vi "Download Web File.vi"(6 "Show File?":bool, 8 "Error In":errorcluster, 9 "timeout (10000)":i32=10000, 10 "Dest Folder":path=path "C:/", 11 "URL":string) -> (0 "Error Out":errorcluster, 1 "body":string, 2 "headers":string, 3 "File Path":path)   [LabVIEW 2021, in "Web.lvlib"]
uses:
  Web.lvlib
  <vilib>/httpClient/LabVIEWHTTPClient.lvlib
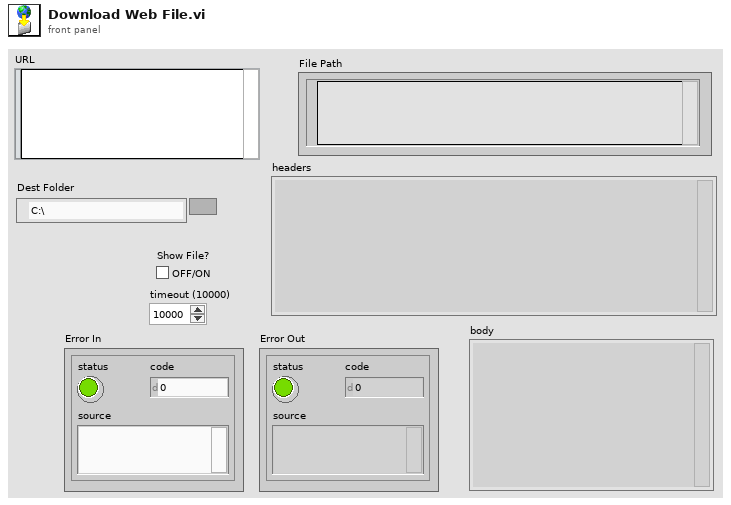
[diagram p1: front panel]
types:
  T1 = typedef "LabVIEWHTTPClient.lvlib/ClientHandle.ctl" = refnum<k1>
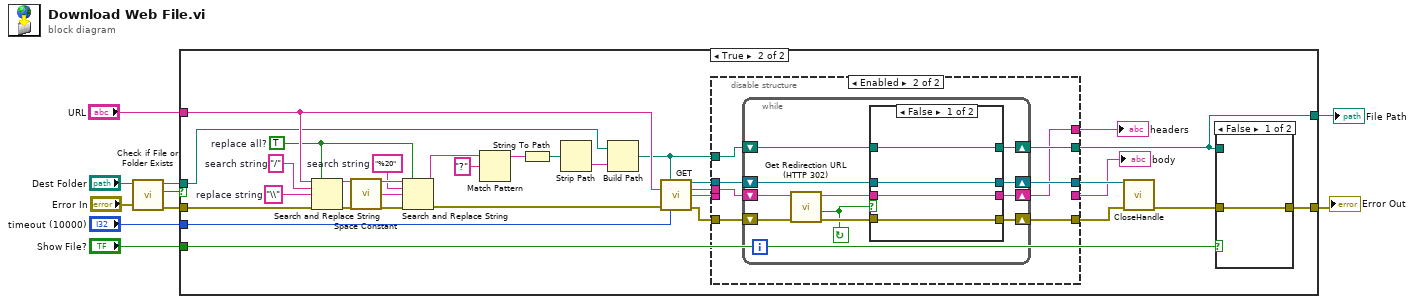
[diagram p0: block diagram]
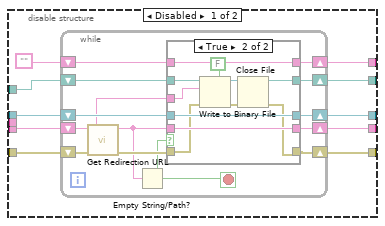
[diagram p3: hidden frame]
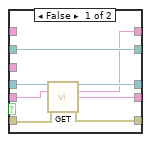
[diagram p4: hidden frame]
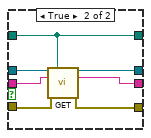
[diagram p5: hidden frame]
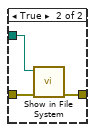
[diagram p6: hidden frame]
diagram:
  n1 = call <vilib>:"Check if File or Folder Exists.vi"("error in (no error)"="Error In", "path"="Dest Folder") -> ("error out"=w8:errorcluster, "file or folder exists?"=w5:bool, "dup path"=w7:path)  [unwired: 7 in]
  n2 = case shown="True" w5 {
    tunnel: "URL" -> [_ w41]
    tunnel: w8 -> [w11 w36]
    tunnel: w7 -> [_ w32]
    tunnel: [w11 w35] -> w2
    tunnel: "Show File?" -> [_ w34]
    tunnel: "timeout (10000)" -> [_ w33]
    tunnel: [_ w18] -> w1
    frame False {
    }
    frame True {
      w24 = "%20"  # search string
      w25 = TRUE  # replace all?
      w39 = "\\"  # replace string
      w40 = "/"  # search string
      n3 = Search and Replace String(replace all?=w25, input string=w41, search string=w40, replace string=w39, error in=w36) -> (result string=w27:string, error out=w29:errorcluster)  [unwired: 3 in, 2 out]
      n4 = call <vilib>:"Space Constant.vi"() -> ("String"=w23:string)
      n5 = Search and Replace String(replace all?=w25, input string=w27, search string=w24, replace string=w23, error in=w29) -> (result string=w26:string, error out=w28:errorcluster)  [unwired: 3 in, 2 out]
      n6 = Match Pattern(string=w26, regular expression="?") -> (before substring=w30:string)  [unwired: 1 in, 3 out]
      n7 = String To Path(string=w30) -> (path=w38:path)
      n8 = Strip Path(path=w38) -> (name=w37:string)  [unwired: 1 out]
      n9 = Build Path(base path=w32, name or relative path=w37) -> (appended path=w14:path)
      n10 = call <vilib>:"GET.vi"("output file"=w14, "url"=w41, "error in (no error)"=w28, "timeout (10000)"=w33) -> ("client handle out"=w20:T1, "headers"=w13:string, "body"=w22:string, "error out"=w21:errorcluster)  [unwired: 8 in]
      n11 = disable-structure shown="Enabled" {
        disable-tunnel: w22 -> [w51 _]
        disable-tunnel: w21 -> [w50 w91]
        disable-tunnel: w20 -> [w49 w90]
        disable-tunnel: [w48 w89] -> w19
        disable-tunnel: [w47 w88] -> w18
        disable-tunnel: [w46 w87] -> w17
        disable-tunnel: [w45 _] -> w16
        disable-tunnel: [w44 w84] -> w15
        disable-tunnel: w14 -> [w43 w86]
        disable-tunnel: w13 -> [_ w85]
        frame Disabled {
          n12 = while {
            shift-right: [w55] -> w46
            shift-left: w50 -> [w64]
            shift-right: [w58] -> w45
            shift-left: w51 -> [w57]
            shift-right: [w62] -> w48
            shift-left: w49 -> [w63]
            shift-right: [w54] -> w47
            shift-left: w43 -> [w56]
            shift-right: [w53] -> w44
            shift-left: "" -> [w52]
            stop <- w59 stop-if-true
            n13 = call "Get Redirection URL.vi"("error in (no error)"=w64, "HTTP GET Body"=w57) -> ("error out"=w61:errorcluster, "Redirection URL"=w60:string)  [unwired: 8 in]
            n14 = Empty String/Path?(string/path=w60) -> (empty?=w59:bool)
            n15 = case shown="True" w59 {
              tunnel: w63 -> [w72 w83]
              tunnel: [w71 w83] -> w62
              tunnel: w61 -> [w70 w74]
              tunnel: w60 -> [w69 w82]
              tunnel: [w68 w82] -> w58
              tunnel: w57 -> [_ w80]
              tunnel: w56 -> [w66 w81]
              tunnel: [w67 w76] -> w55
              tunnel: [w66 w75] -> w54
              tunnel: [w65 w73] -> w53
              tunnel: w52 -> [_ w73]
              frame False {
                n16 = call <vilib>:"GET.vi"("client handle"=w72, "url"=w69, "error in (no error)"=w70) -> ("client handle out"=w71:T1, "headers"=w65:string, "body"=w68:string, "error out"=w67:errorcluster)  [unwired: 9 in]
              }
              frame True {
                n17 = Write to Binary File(file (use dialog)=w81, data=w80, error in=w74, 5:FALSE ("prepend array or string size? (T)")) -> (refnum out=w78:refnum<file>, error out=w77:errorcluster)  [unwired: 2 in, 1 out]
                n18 = Close File(refnum=w78, error in=w77) -> (path=w75:path, error out=w76:errorcluster)
              }
            }
          }
        }
        frame Enabled {
          n19 = while {
            shift-right: [w94] -> w87
            shift-left: w91 -> [w102]
            shift-right: [w97] -> w84
            shift-left: w85 -> [w96]
            shift-right: [w100] -> w89
            shift-left: w90 -> [w101]
            shift-right: [w93] -> w88
            shift-left: w86 -> [w95]
            stop <- w92 continue-if-true
            n20 = call "Get Redirection URL (HTTP 302).vi"("error in (no error)"=w102, "HTTP GET Header"=w96) -> ("error out"=w99:errorcluster, "redirection"=w92:bool, "Redirection URL"=w98:string)  [unwired: 7 in]
            n21 = case shown="False" w92 {
              tunnel: w101 -> [w106 w113]
              tunnel: [w106 w112] -> w100
              tunnel: w99 -> [w103 w111]
              tunnel: w98 -> [w105 w110]
              tunnel: [w105 w107] -> w97
              tunnel: w95 -> [w104 w108]
              tunnel: [w103 w109] -> w94
              tunnel: [w104 w108] -> w93
              frame False {
              }
              frame True {
                n22 = call <vilib>:"GET.vi"("client handle"=w113, "output file"=w108, "url"=w110, "error in (no error)"=w111) -> ("client handle out"=w112:T1, "headers"=w107:string, "error out"=w109:errorcluster)  [unwired: 8 in, 1 out]
              }
            }
          }
        }
      }
      "headers" <- w15
      "body" <- w16
      n23 = call <vilib>:"CloseHandle.vi"("client handle"=w19, "error in (no error)"=w17) -> ("error out"=w12:errorcluster)  [unwired: 13 in]
      n24 = case shown="False" w34 {
        tunnel: w18 -> [_ w117]
        tunnel: w12 -> [w114 w116]
        tunnel: [w114 w115] -> w35
        frame False {
        }
        frame True {
          n25 = call <vilib>:"Show in File System.vi"("error in (no error)"=w116, "file or directory path"=w117) -> ("error out"=w115:errorcluster)  [unwired: 9 in]
        }
      }
    }
  }
  "Error Out" <- w2
  "File Path" <- w1
